vi "WriteAttributesTest.vi"(3 "device name":string="tango/tangotest/1") -> ()   [LabVIEW 2009]
uses:
  tango_lv8/tango_vi.llb/fromStringScalar.vi
  tango_lv8/tango_vi.llb/fromShortScalar.vi
  tango_lv8/tango_vi.llb/fromLongScalar.vi
  tango_lv8/tango_vi.llb/fromDoubleScalar.vi
panel:
  out "error code":i32
  out "error stack":string[](array[string])
  out "success":bool
  in  "value":dbl=123.456
  in  "attribute name":string="double_scalar"
  in  "value":i32=32768
  in  "attribute name":string="long_scalar"
  in  "value":i16=256
  in  "attribute name":string="short_scalar"
  in  "value":string="This is the write value..."
  in  "attribute name":string="string_scalar"
  # "TANGO  Binding for LabVIEW - WriteAttributes example"
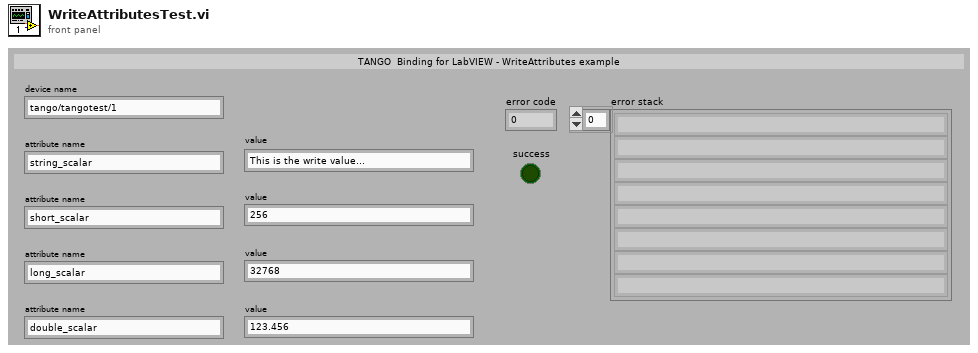
[diagram p1: front panel]
types:
  T1 = cluster{"device name":string, "attribute name":string, "quality value":i16, "quality string":string, "timestamp":dbl, "dim. x":i32, "dim. y":i32, "value":u8[], "error code":i32, "error stack":string[], "data type":enum16{"SCA_STATE", "SCA_STRING", "SPE_STRING", "IMG_STRING", "SCA_BOOLEAN", "SPE_BOOLEAN", "IMG_BOOLEAN", "SCA_UCHAR", "SPE_UCHAR", "IMG_UCHAR", "SCA_SHORT", "SPE_SHORT", "IMG_SHORT", "SCA_USHORT", "SPE_USHORT", "IMG_USHORT", "SCA_LONG", "SPE_LONG", "IMG_LONG", "SCA_ULONG", "SPE_ULONG", "IMG_ULONG", "SCA_FLOAT", "SPE_FLOAT", "IMG_FLOAT", "SCA_DOUBLE", "SPE_DOUBLE", "IMG_DOUBLE", "UNKNOWN_TYPE"}}
  T2 = cluster{"device name":string, "attribute name":string, "quality value":i16, "quality string":string, "timestamp":dbl, "dim. x":i32, "dim. y":i32, "value":u8[], "error code":i32, "error stack":string[], "data type":enum16{"SCA_STATE", "SCA_STRING", "SPE_STRING", "IMG_STRING", "SCA_BOOLEAN", "SPE_BOOLEAN", "IMG_BOOLEAN", "SCA_UCHAR", "SPE_UCHAR", "IMG_UCHAR", "SCA_SHORT", "SPE_SHORT", "IMG_SHORT", "SCA_USHORT", "SPE_USHORT", "IMG_USHORT", "SCA_LONG", "SPE_LONG", "IMG_LONG", "SCA_ULONG", "SPE_ULONG", "IMG_ULONG", "SCA_FLOAT", "SPE_FLOAT", "IMG_FLOAT", "SCA_DOUBLE", "SPE_DOUBLE", "IMG_DOUBLE", "UNKNOWN_TYPE"}}[]
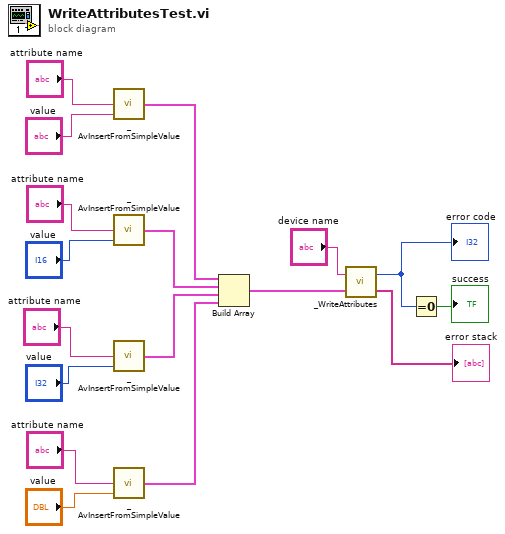
[diagram p0: block diagram]
diagram:
  n1 = call-poly "_AvInsertFromSimpleValue.vi"("value"="value", "attribute name"="attribute name") -> ("attribute value"=w10:T1)  [unwired: 1 in]
  n2 = call-poly "_AvInsertFromSimpleValue.vi"("value"="value", "attribute name"="attribute name") -> ("attribute value"=w8:T1)  [unwired: 1 in]
  n3 = call-poly "_AvInsertFromSimpleValue.vi"("value"="value", "attribute name"="attribute name") -> ("attribute value"=w5:T1)  [unwired: 1 in]
  n4 = call-poly "_AvInsertFromSimpleValue.vi"("value"="value", "attribute name"="attribute name") -> ("attribute value"=w2:T1)  [unwired: 1 in]
  n5 = Build Array(w10, w8, w5, w2) -> (w9:T2)
  n6 = call "_WriteAttributes.vi"("values"=w9, "device name"="device name") -> ("error stack"=→"error stack":string[], "error code"=w16:i32)
  "error code" <- w16
  n7 = Equal To 0?(x=w16) -> (x = 0?=→"success":bool)
